vi "Script_Timing_List_From_Directory.vi"(7 "Refnum LstDér":refnum<vi>, 8 "error in (no error)":errorcluster, 9 "Timing Scripts File Filter":string, 10 "Timing Scripts Path":path, 11 "Refnum Tabl":refnum<vi>) -> (0 "error out":errorcluster, 1 "List of Scripts":string[](array[string]), 2 "Table of Scripts":string[](array[string]), 3 "Refnum Tabl Out":refnum<vi>, 5 "Refnum LstDér Out":refnum<vi>)   [LabVIEW 2017]
panel:
  out "String of Scripts":string
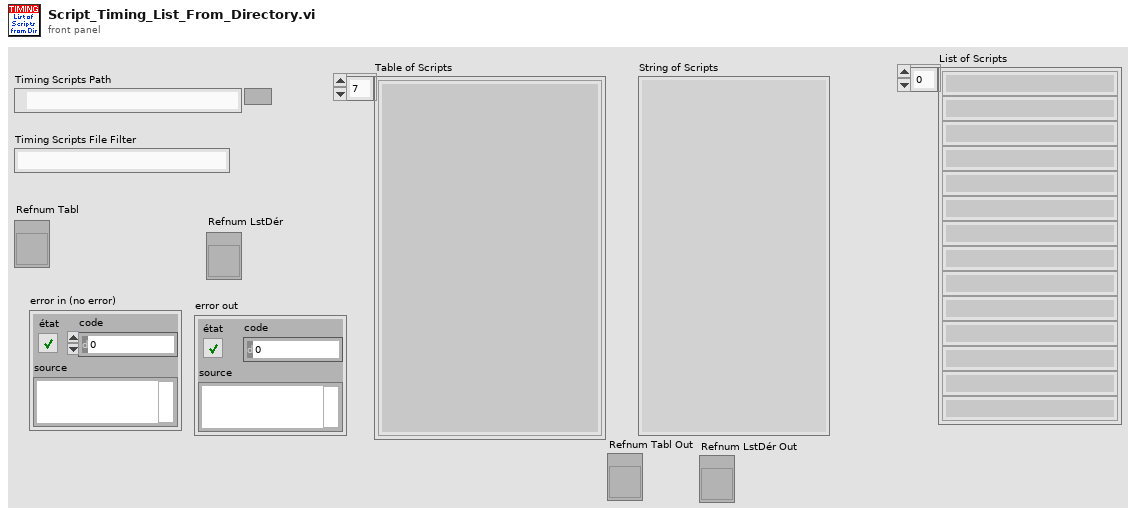
[diagram p1: front panel]
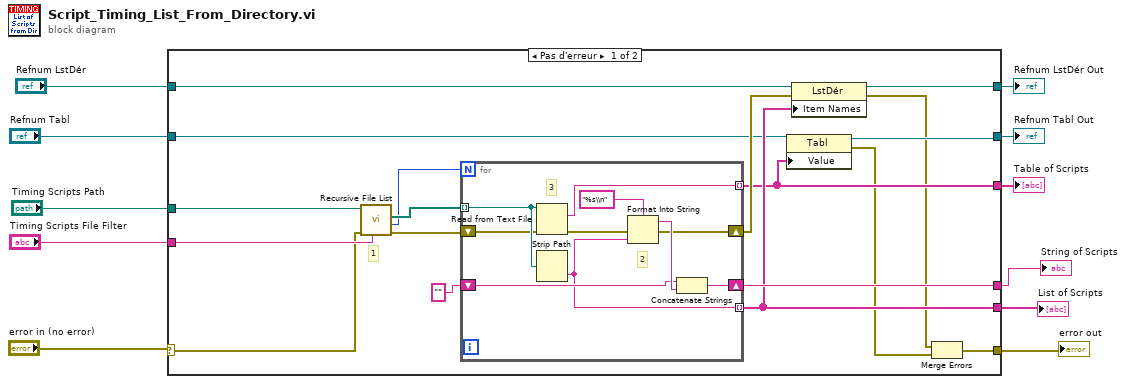
[diagram p0: block diagram]
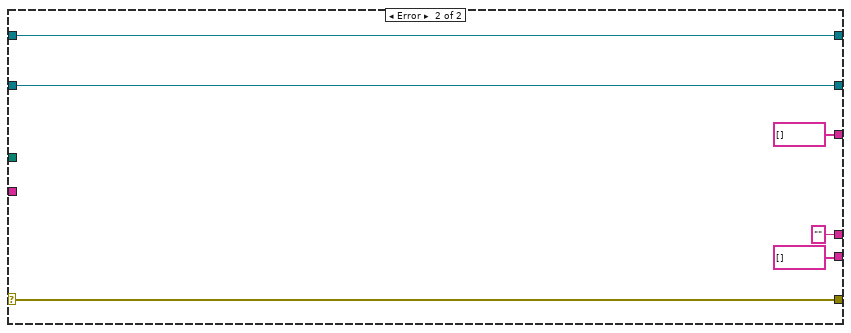
[diagram p2: hidden frame]
diagram:
  n1 = case shown="Pas d'erreur" "error in (no error)" {
    selector: "error in (no error)" -> [w23 w45]
    tunnel: "Timing Scripts Path" -> [w25 _]
    tunnel: "Timing Scripts File Filter" -> [w24 _]
    tunnel: [w16 string[] []] -> w8
    tunnel: [w22 ""] -> w7
    tunnel: [w12 w45] -> w6
    tunnel: [w20 string[] []] -> w5
    tunnel: "Refnum LstDér" -> [w21 w41]
    tunnel: [w19 w41] -> w3
    tunnel: "Refnum Tabl" -> [w17 w40]
    tunnel: [w15 w40] -> w1
    frame No Error {
      # "1"
      n2 = call <vilib>:"Recursive File List.vi"("pattern"=w24, "error in (no error)"=w23, "Folder Path"=w25) -> ("error out"=w26:errorcluster, "Number of Files"=w27:i32, "All Files in Dir"=w29:path[])  [unwired: 4 in, 2 out]
      n3 = for {
        N: w27 -> [_]
        tunnel: w29 -> [w38] mode=indexing
        tunnel: [w39] -> w16 mode=indexing
        shift-right: [w35] -> w22
        shift-left: "" -> [w34]
        shift-right: [w31] -> w18
        shift-left: w26 -> [w33]
        tunnel: [w30] -> w20 mode=indexing
        # "3"
        # "2"
        n4 = Read from Text File(file (use dialog)=w38, error in=w33) -> (text=w39:string, error out=w32:errorcluster)  [unwired: 2 in, 2 out]
        n5 = Strip Path(path=w38) -> (name=w30:string)  [unwired: 1 out]
        n6 = Format Into String(format string="%s\\n" ("chaîne de format"), error in=w32, w30) -> (resulting string=w36:string, error out=w31:errorcluster)  [unwired: 1 in]
        n7 = Concatenate Strings(w34, w36) -> (w35:string)
      }
      n8 = property class="Tabl"(reference=w17, "Value"=w16) -> (reference out=w15:refnum<vi>, error out=w14:errorcluster)  [unwired: 1 in]
      n9 = property class="LstDér"(reference=w21, error in=w18, "Item Names"=w20) -> (reference out=w19:refnum<vi>, error out=w13:errorcluster)
      n10 = Merge Errors(w13, w14) -> (w12:errorcluster)
    }
    frame Error {
    }
  }
  "error out" <- w6
  "Table of Scripts" <- w8
  "String of Scripts" <- w7
  "List of Scripts" <- w5
  "Refnum LstDér Out" <- w3
  "Refnum Tabl Out" <- w1
